vi "Set Config.vi"(8 "error in (no error)":errorcluster, 9 "Config Data":variant, 11 "CAP-USB-1 in":refnum<class "CAP-USB-1.lvclass">) -> (0 "error out":errorcluster, 3 "CAP-USB-1 out":refnum<class "CAP-USB-1.lvclass">)   [LabVIEW 2014, in "CAP-USB-1.lvlib" / "CAP-USB-1.lvclass"]
uses:
  CAP-USB-1.lvclass
  CAP-USB-1.lvclass/CAP-USB-1.ctl
  DriverMasterSync/build/DriverMasterSync.lvlibp/Modules/HAL/DriverMasterSync/DriverMasterSyncClass/DriverMasterSync.lvclass
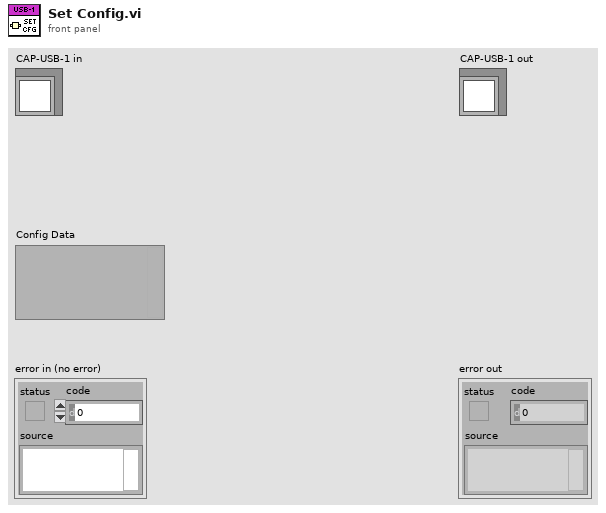
[diagram p1: front panel]
types:
  T1 = typedef "DriverMasterSync.lvlibp/HAL Config Data.ctl" = cluster{"HWSync Index":u32, "Driver Name":string, "Channel Mask":u64}
  T2 = cluster{"VISA resource name":refnum<visa-resource-name>}
  T3 = cluster{"Transductores":u64, "Delay uS":i32, "Delay uS Seq":i32, "Num de tramas":u32, "Tamaño Script":i32, "Orden Transd":u64, "Pulsos encoder":u16, "Offset":sgl[], "Gain":sgl[], "Reduccion":sgl, "Proteccion T":u64}
  T4 = cluster{"Promedio Transd":sgl[], "Tolerancia":sgl, "Test Ok":bool[], "Muestras Diag. Cycle":u32, "Tolerancia Cycle":sgl}
  T5 = cluster{"Channel Mask":u64, "Connection Data":cluster{"VISA resource name":refnum<visa-resource-name>}, "Config Data":cluster{"Transductores":u64, "Delay uS":i32, "Delay uS Seq":i32, "Num de tramas":u32, "Tamaño Script":i32, "Orden Transd":u64, "Pulsos encoder":u16, "Offset":sgl[], "Gain":sgl[], "Reduccion":sgl, "Proteccion T":u64}, "Diagnostic Data":cluster{"Promedio Transd":sgl[], "Tolerancia":sgl, "Test Ok":bool[], "Muestras Diag. Cycle":u32, "Tolerancia Cycle":sgl}, "Comandos":cluster{"Salidas":bool[]}}
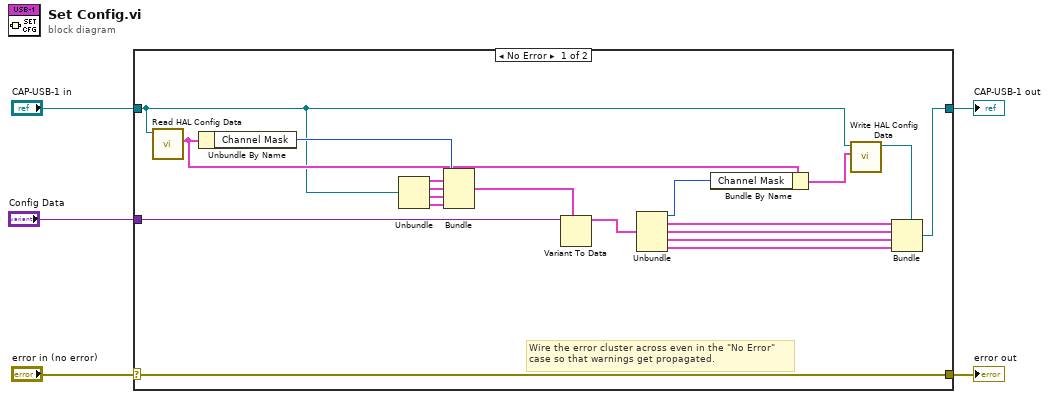
[diagram p0: block diagram]
diagram:
  n1 = case shown="No Error" "error in (no error)" {
    selector: "error in (no error)" -> [w24 w26]
    tunnel: [w24 w26] -> w4
    tunnel: [w22 w25] -> w2
    tunnel: "CAP-USB-1 in" -> [w17 w25]
    tunnel: "Config Data" -> [w23 _]
    frame No Error {
      # "Wire the error cluster across even in the \"No Error\"\ncase so that warnings get propagated."
      n2 = call "Read HAL Config Data.vi"("DriverMasterSync in"=w17) -> ("HAL Config Data"=w19:T1)  [unwired: 8 in, 2 out]
      n3 = Unbundle By Name(w19) -> ("Channel Mask"=w21:u64)
      n4 = Unbundle(w17) -> (w16:T2, w15:T3, w14:T4, w13:cluster{"Salidas":bool[]})
      n5 = Bundle("Channel Mask"=w21, "Connection Data"=w16, "Config Data"=w15, "Diagnostic Data"=w14, "Comandos"=w13) -> (w12:T5)  [unwired: 1 in]
      n6 = Variant To Data(type=w12, Variant=w23) -> (data=w11:T5)  [unwired: 1 in, 1 out]
      n7 = Unbundle(w11) -> ("Channel Mask"=w10:u64, "Connection Data"=w9:T2, "Config Data"=w8:T3, "Diagnostic Data"=w7:T4, "Comandos"=w6:cluster{"Salidas":bool[]})
      n8 = Bundle By Name(cluster=w19, "Channel Mask"=w10) -> (w18:T1)
      n9 = call "Write HAL Config Data.vi"("HAL Config Data"=w18, "DriverMasterSync in"=w17) -> ("DriverMasterSync out"=w20:refnum<class "CAP-USB-1.lvclass">)  [unwired: 8 in, 1 out]
      n10 = Bundle(cluster=w20, w9, w8, w7, w6) -> (w22:refnum<class "CAP-USB-1.lvclass">)
    }
    frame Error {
    }
  }
  "error out" <- w4
  "CAP-USB-1 out" <- w2
